vi "Fault Handling.vi"(8 "error in (no error)":errorcluster, 10 "FaultCode":i32, 11 "Ignition in":refnum<class "Ignition.lvclass">) -> (0 "error out":errorcluster, 2 "Fault codes":cluster{"Bit":string, "Description":string}[](array[cluster]), 3 "Ignition out":refnum<class "Ignition.lvclass">)   [LabVIEW 2021]
uses:
  Ignition.lvclass
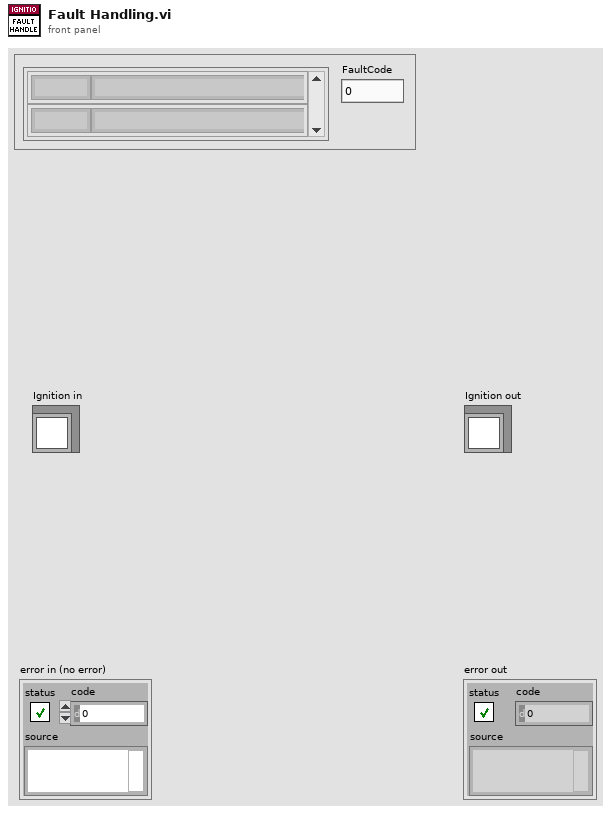
[diagram p1: front panel]
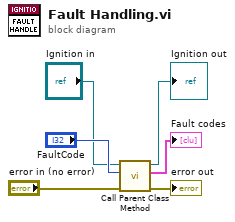
[diagram p0: block diagram]
diagram:
  n1 = call-parent "Call Parent Class Method"("error in (no error)"="error in (no error)", "FaultCode"="FaultCode", "OPC UA in"="Ignition in") -> ("error out"=→"error out":errorcluster, "Fault codes"=→"Fault codes":cluster{"Bit":string, "Description":string}[], "OPC UA out"=→"Ignition out":refnum<class "Ignition.lvclass">)  [unwired: 6 in]
